vi "SubPanel_PowerConfiguration_Rev11_v4.vi"(8 "error in":errorcluster, 10 "VISAPowerInfoInputArray":T2(array[cluster]), 11 "DCPowerInformationClusterArray_Input":T1(array[cluster])) -> (0 "error out":errorcluster, 2 "VISAPowerInfoOutputArray":T2(array[cluster]), 3 "DCPowerInformationClusterArray_Output":T1(array[cluster]))   [LabVIEW 2019]
uses:
  Controls/PlotColorArray.ctl
panel:
  out "Current Numeric (A)":dbl[][](array[numeric])
  out "Voltage Numeric (V)":dbl[][](array[numeric])
  out "Voltage Waveform Array":waveform(dbl)[](graph)
  out "Current Waveform Array":waveform(dbl)[](graph)
  out "Supplies Updated?":bool
  out "DCPowerInformationClusterArray":T1(array[cluster])
  in  "Update Changes (MUST HAVE ACTIVE CHANNEL SELECTED FOR CHANGES TO BE APPLIED)":bool
  out "VISAPowerInformationClusterArray":T2(array[cluster])
  out "VISAPowerInformationClusterOutput":T3(array[cluster])
  in  "VISAPowerInformationClusterInput":T3(array[cluster])
  in  "Exit SubVI":bool
  in  "Instrument Cards (Must Reconfigure if you add new cards or change the names in NI Max)":T4(tab)
  in  "VISA resource name":refnum<visa-resource-name>
  in  "Apply Power Settings":bool
  out "POWER STATUS":bool
  in  "POWER ON":bool
  in  "Voltage Channel 1":dbl
  in  "Voltage Channel 2":dbl
  in  "Voltage Channel 3":dbl
  in  "Current Limit Channel 1":dbl
  in  "Current Limit Channel 2":dbl
  in  "Current Limit Channel 3":dbl
  out "Parameter Configuration Echo":string[][](array[string])
  out "Configuration Echo":string
  in  "Which Channels to Parallelize":u16(ring) items=["I1+I2", "ALL", "I2+I3"]
  in  "Combination Scheme":u16(ring) items=["OFF", "SERIES", "PARALLEL"]
  in  "voltage level channel 0":dbl format="%.6p"
  in  "voltage level channel 1":dbl format="%.6p"
  in  "voltage level channel 2":dbl format="%.6p"
  in  "voltage level channel 3":dbl format="%.6p"
  in  "voltage level channel 4":dbl format="%.6p"
  in  "voltage level channel 5":dbl format="%.6p"
  in  "voltage level channel 6":dbl format="%.6p"
  in  "voltage level channel 7":dbl format="%.6p"
  in  "voltage level channel 8":dbl format="%.6p"
  in  "voltage level channel 9":dbl format="%.6p"
  in  "voltage level channel 10":dbl format="%.6p"
  in  "voltage level channel 11":dbl format="%.6p"
  in  "voltage level channel 12":dbl format="%.6p"
  in  "voltage level channel 13":dbl format="%.6p"
  in  "voltage level channel 14":dbl format="%.6p"
  in  "voltage level channel 15":dbl format="%.6p"
  in  "voltage level channel 16":dbl format="%.6p"
  in  "voltage level channel 17":dbl format="%.6p"
  in  "voltage level channel 18":dbl format="%.6p"
  in  "voltage level channel 19":dbl format="%.6p"
  in  "voltage level channel 20":dbl format="%.6p"
  in  "voltage level channel 21":dbl format="%.6p"
  in  "voltage level channel 22":dbl format="%.6p"
  in  "voltage level channel 23":dbl format="%.6p"
  in  "Active Channel 0":bool
  in  "Active Channel 1":bool
  in  "Active Channel 2":bool
  in  "Active Channel 3":bool
  in  "Active Channel 4":bool
  in  "Active Channel 5":bool
  in  "Active Channel 6":bool
  in  "Active Channel 7":bool
  in  "Active Channel 8":bool
  in  "Active Channel 9":bool
  in  "Active Channel 10":bool
  in  "Active Channel 11":bool
  in  "Active Channel 12":bool
  in  "Active Channel 13":bool
  in  "Active Channel 14":bool
  in  "Active Channel 15":bool
  in  "Active Channel 16":bool
  in  "Active Channel 17":bool
  in  "Active Channel 18":bool
  in  "Active Channel 19":bool
  in  "Active Channel 20":bool
  in  "Active Channel 21":bool
  in  "Active Channel 22":bool
  in  "Active Channel 23":bool
  in  "Channel Name 0":string="NULL0"
  in  "Channel Name 1":string="NULL1"
  in  "Channel Name 2":string="NULL2"
  in  "Channel Name 3":string="NULL3"
  in  "Channel Name 4":string="NULL4"
  in  "Channel Name 5":string="NULL5"
  in  "Channel Name 6":string="NULL6"
  in  "Channel Name 7":string="NULL7"
  in  "Channel Name 8":string="NULL8"
  in  "Channel Name 9":string="NULL9"
  in  "Channel Name 10":string="NULL10"
  in  "Channel Name 11":string="NULL11"
  in  "Channel Name 12":string="NULL12"
  in  "Channel Name 13":string="NULL13"
  in  "Channel Name 14":string="NULL14"
  in  "Channel Name 15":string="NULL15"
  in  "Channel Name 16":string="NULL16"
  in  "Channel Name 17":string="NULL17"
  in  "Channel Name 18":string="NULL18"
  in  "Channel Name 19":string="NULL19"
  in  "Channel Name 20":string="NULL20"
  in  "Channel Name 21":string="NULL21"
  in  "Channel Name 22":string="NULL22"
  in  "Channel Name 23":string="NULL23"
  in  "Apply Power Settings":bool
  in  "Aperture Time (s)":dbl=0.0001
  in  "Measure Record Length":i32=1000000
  in  "current limit (A)":dbl=0.05
  out "All Channel Numbers Array":string[](array[string])=["0", "1", "2", "3", "4", "5", "6", "7", "8", "9", "10", "11", "12", "13", "14", "15", "16", "17", "18", "19", "20", "21", "22", "23"]
  out "Active Channels Indicator":bool[](array[boolean])
  out "Voltage Array":dbl[](array[numeric])
  out "Active Channel Numbers Array":string[](array[string])
  out "Active Channel Voltage Array":dbl[](array[numeric])
  out "Active Channel Names Array":string[](array[string])
  in  "voltage level channel 0":dbl=1.0 format="%.6p"
  in  "Active Channel 0":bool
  in  "Apply Power Settings":bool
  in  "Channel Name 0":string="NULL_0_slot16"
  out "Active Channel Voltage Array":dbl[](array[numeric])
  out "Active Channels Indicator":bool[](array[boolean])
  out "Voltage Array":dbl[](array[numeric])=[1.0]
  out "Active Channel Names Array":string[](array[string])
  out "Active Channel Numbers Array":string[](array[string])
  out "All Channel Numbers Array":string[](array[string])=["0"]
  in  "current limit (A)":dbl=3.0
  in  "Measure Record Length":i32=1000000
  in  "Aperture Time (s)":dbl=0.001
  in  "Apply Power Settings":bool
  in  "Aperture Time (s)":dbl=0.001
  in  "Measure Record Length":i32=1000000
  in  "current limit (A)":dbl=3.0
  in  "Active Channel 0":bool
  in  "voltage level channel 24":dbl=2.0 caption="voltage level channel 0" format="%.6p"
  in  "Channel Name 0":string="NULL_0_slot_16"
  out "Active Channel Names Array":string[](array[string])
  out "Active Channel Voltage Array":dbl[](array[numeric])
  out "Active Channel Numbers Array":string[](array[string])
  out "Voltage Array":dbl[](array[numeric])=[2.0]
  out "Active Channels Indicator":bool[](array[boolean])
  out "All Channel Numbers Array":string[](array[string])=["0"]
  out "Active Channel Names Array":string[](array[string])
  out "Active Channel Voltage Array":dbl[](array[numeric])
  out "Active Channel Numbers Array":string[](array[string])
  out "Voltage Array":dbl[](array[numeric])=[3.0]
  out "All Channel Numbers Array":string[](array[string])=["0"]
  out "Active Channels Indicator":bool[](array[boolean])
  in  "voltage level channel 25":dbl=3.0 caption="voltage level channel 0" format="%.6p"
  in  "Active Channel 0":bool
  in  "Channel Name 0":string="NULL_0_slot16"
  in  "Apply Power Settings":bool
  in  "Aperture Time (s)":dbl=0.001
  in  "Measure Record Length":i32=1000000
  in  "current limit (A)":dbl=3.0
  out "DCPowerInformationClusterOutput":T5(array[cluster])
  in  "DCPowerInformationClusterInput":T5(array[cluster])
  in  "ColorPalette":T6=[16711686, 65351, 8978420, 14474240, 16139007, 16752640, 8958719, 16758973, 16777215, 46792, 11992992, 12961221, 16763690, 12600063, 16711835, 2953983, 40796, 13111296, 13352613, 9221011, 12964076, 12819897, 65442, 16776704, 14540253, 16740729, 10658047, 10813344, 16753521, 13413843, 8691115, 10339240, 14401205, 16746704, 7467519, 16775978, 13872558, 11387603, 13354405, 10420227, 13107364, 4060, 35208, 11817216, 7566080, 40796, 7539456, 2837073, 6372186, 7499083, 10648702, 16757152]
  # "Background Information (Important)\nThis subvi has tabs that allow you to configure different power instruments. There are two options: VISA instruments or DC Power instruments. DC Power instruments are inside of the tester, visa instruments are external. If DCPower instruments are switched out, they will need to be reconfigured within the backend of this code (instructions pending). You are able to identify which channels you want to active, their individual voltage levels and the desired \"name\" of the channel (i.e. if you want channel 0 to be known at the \"ADMV1013_3p3V\" or \"GoodEnough\", you write it here). For the entire instrument, you can determine its capture rate (aperture time) or the current limit. I advise you do NOT alter the \"Measure Record Length\" as this is only if there are issues with the program. Shouldn't ever exceed this value. You apply the settings and they will be echoed back in each tab along with the array above. Multiple instruments can be configured and will show up as separate array elements\n\n\nInstructions (More Important):\n\nSelect instrument of interest (VISA KEITHLEY 2230G-30-6, PXIe-4163, and PXIe-4139 are the ones currently available). \n\n\nFOR DCPOWER INSTRUMENTS (PXI or PXIe)\n\nPress \"Active Channel #\" to select which channels you want to have power applied \n\nType in voltage level in \"Voltage level channel #\"\n\nType in desired channel name in \"Channel Name #\"\n\nType the measurement speed (suggest .0001) in aperture time\n\nType the current limit in \"current limit\"\n\nPress \"Apply Power Settings\" and review the echoed outputs within the tab and in the instrument array above the tabs.\n\nRepeat this process for other instruments\n\n\n\nFOR VISA INSTRUMENTS (NOT PXI or PXIe), note that it is case by case for instruments\n\nSelect resource name (you must know which one it is)\n\nPower on device if using it\n\nApply voltage settings \n\nApply current limits for each channel\n\nSelect which channels you will parallelize if at all\n\nSelect which combination scheme you will apply: OFF (individual channels), SERIES (Channel 1 and 2 in series), PARALLEL (I1 + I2, ALL, I2 + I3)\n\nFOR COMBINATIONS: for a combination scheme you choose, you only apply changes to the first channel of each. example: if you make the system series configuration, you only type you voltage information (i.e. 60V) into channel 1 and the current limit information into channel 1 but channel 3 is still independent of these\n\n\nPress \"Apply Powe Settings\" when complete\n\nReview the echoed values along with the instrument array above"
  # "All Voltage Level Channels are in Volts"
  # "Don't press enter when typing in strings. Just click out of it"
  # "Don't press enter when typing in strings. Just click out of it"
  # "Don't press enter when typing in strings. Just click out of it"
  # "Don't press enter when typing in strings. Just click out of it"
  # "Don't press enter when typing in strings. Just click out of it"
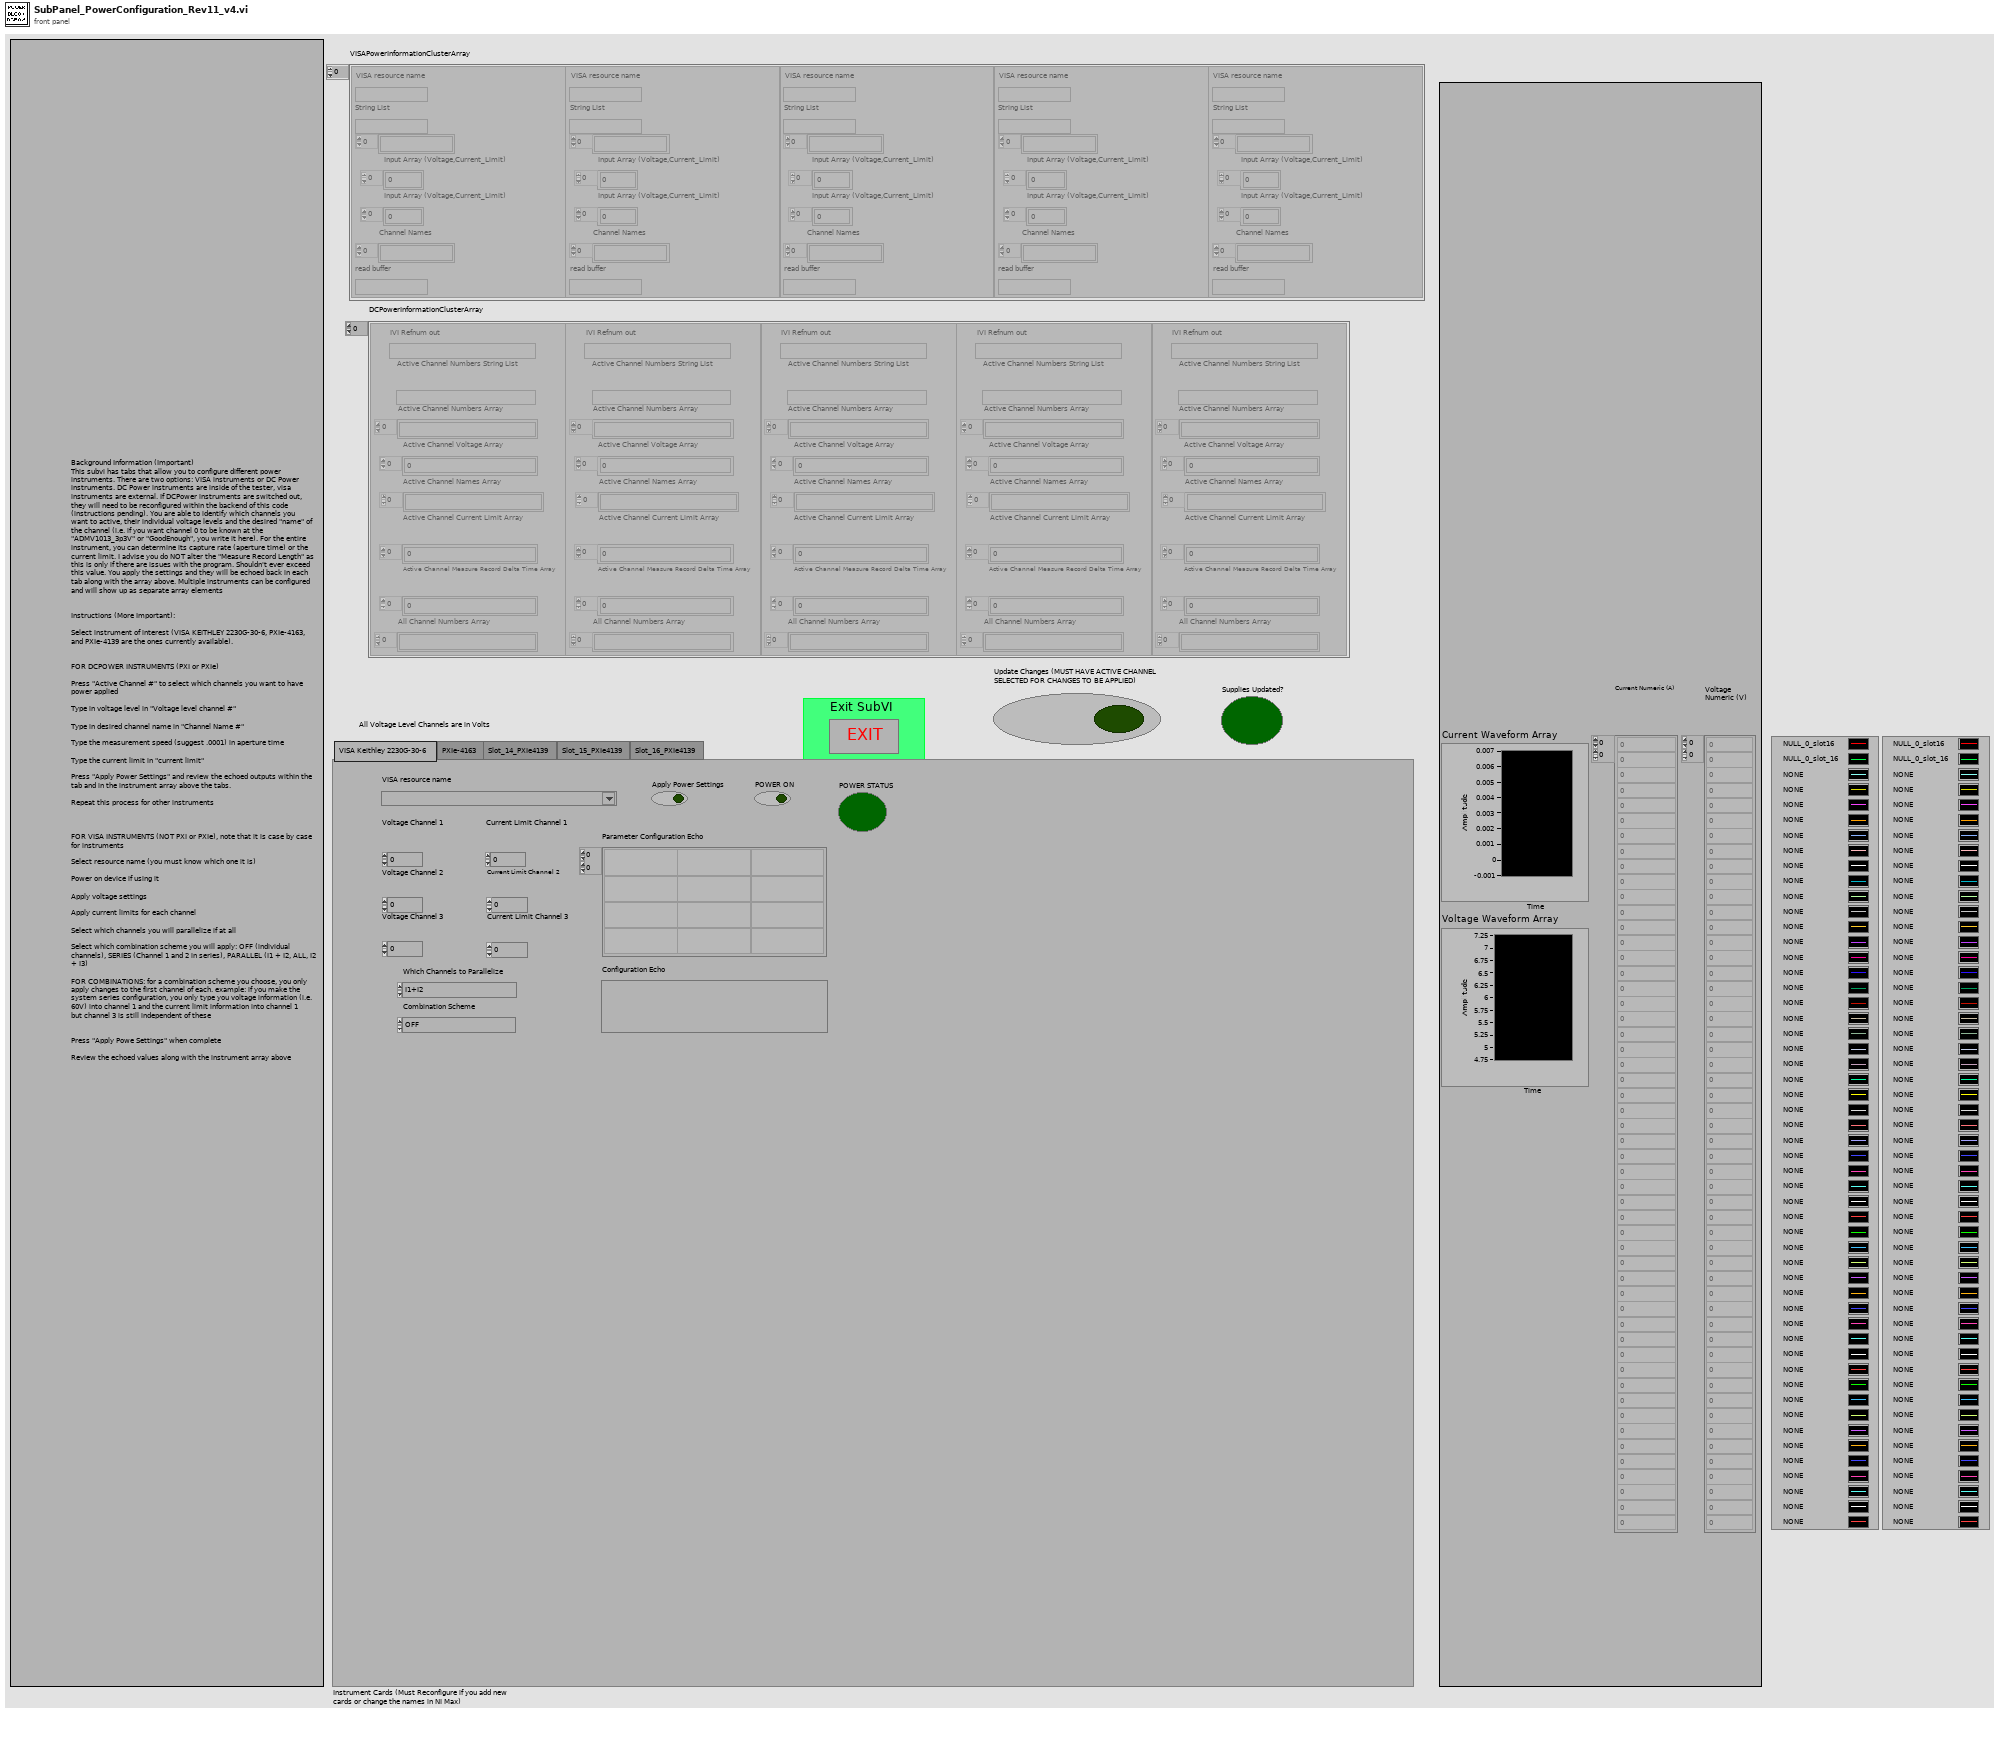
[diagram p1: front panel]
types:
  T1 = cluster{"IVI Refnum out":refnum<k15>, "Active Channel Numbers String List":string, "Active Channel Numbers Array":string[], "Active Channel Voltage Array":dbl[], "Active Channel Names Array":string[], "Active Channel Current Limit Array":dbl[], "Active Channel Measure Record Delta Time Array":dbl[], "All Channel Numbers Array":string[]}[]
  T2 = cluster{"VISA resource name":refnum<visa-resource-name>, "String List":string, string[], "Input Array (Voltage,Current_Limit)":dbl[], "Input Array (Voltage,Current_Limit)":dbl[], "Channel Names":string[], "read buffer":string}[]
  T3 = cluster{"VISA resource name":refnum<visa-resource-name>, "String List":string, string[], "Input Array (Voltage,Current_Limit)":dbl[], "Input Array (Voltage,Current_Limit)":dbl[], "Channel Names":string[]}[]
  T4 = enum32{"VISA Keithley 2230G-30-6", "PXIe-4163", "Slot_14_PXIe4139", "Slot_15_PXIe4139", "Slot_16_PXIe4139"}
  T5 = cluster{"instrument handle out":refnum<k15>, string, string[], dbl[], string[]}[]
  T6 = typedef "PlotColorArray.ctl" = u32[]
  T7 = cluster{"instrument handle out":refnum<k15>, string, string[], dbl[], string[], "Current Limit Output Array":dbl[], dbl[]}[]
  T8 = cluster{"IVI Refnum out":refnum<k15>, "Active Channel Numbers String List":string, "Active Channel Numbers Array":string[], "Active Channel Voltage Array":dbl[], "Active Channel Names Array":string[], "Active Channel Current Limit Array":dbl[], "Active Channel Measure Record Delta Time Array":dbl[], "All Channel Numbers Array":string[]}
  T9 = cluster{"IVI Refnum out":refnum<k15>, string, "voltage level channel 23":dbl, "Channel Name 23":string, "Current Limit":dbl, "Measure Record dt":dbl, string}[]
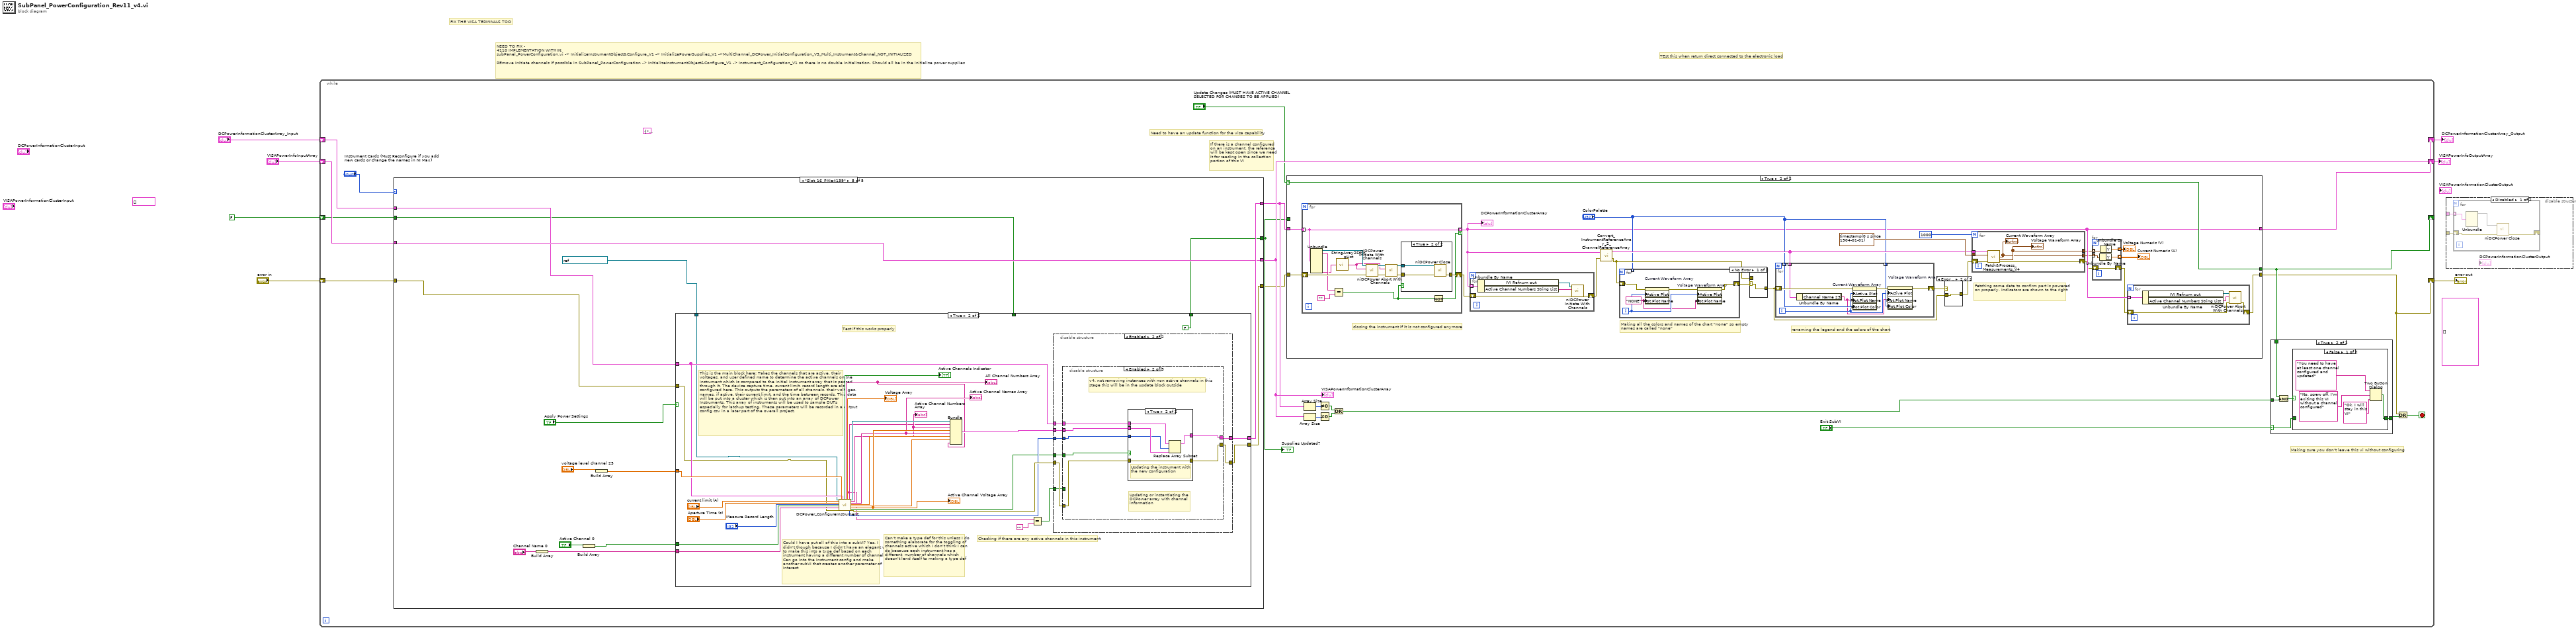
[diagram p0: block diagram]
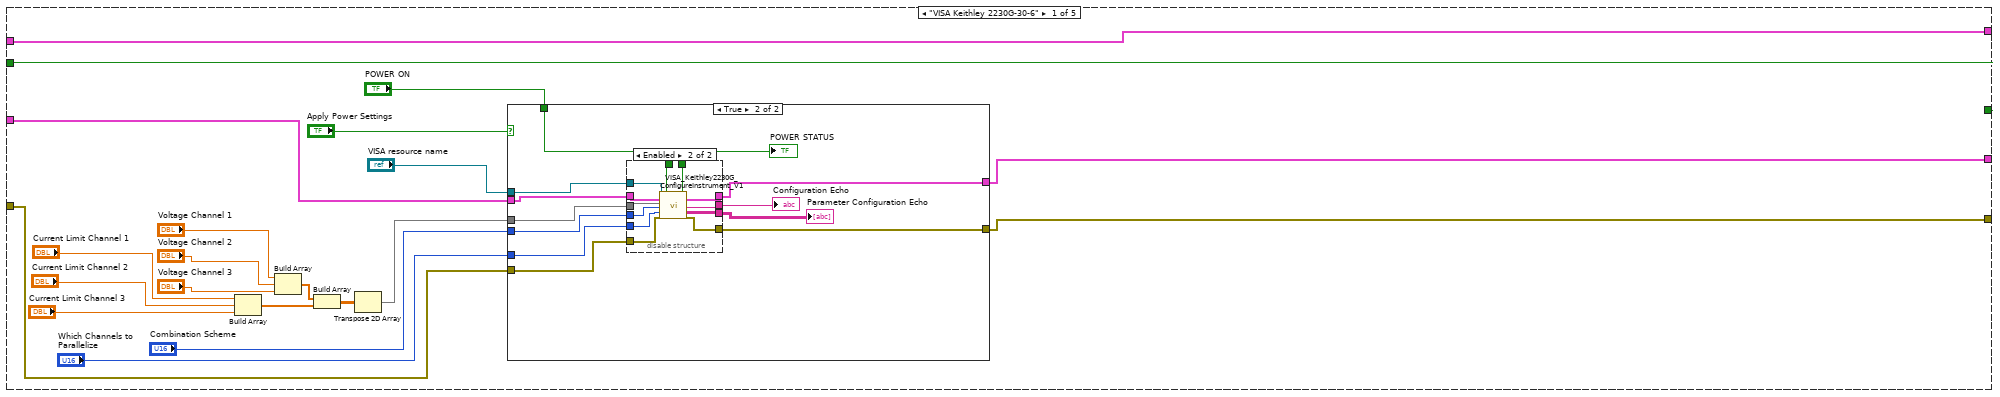
[diagram p9: hidden frame]
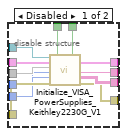
[diagram p11: hidden frame]
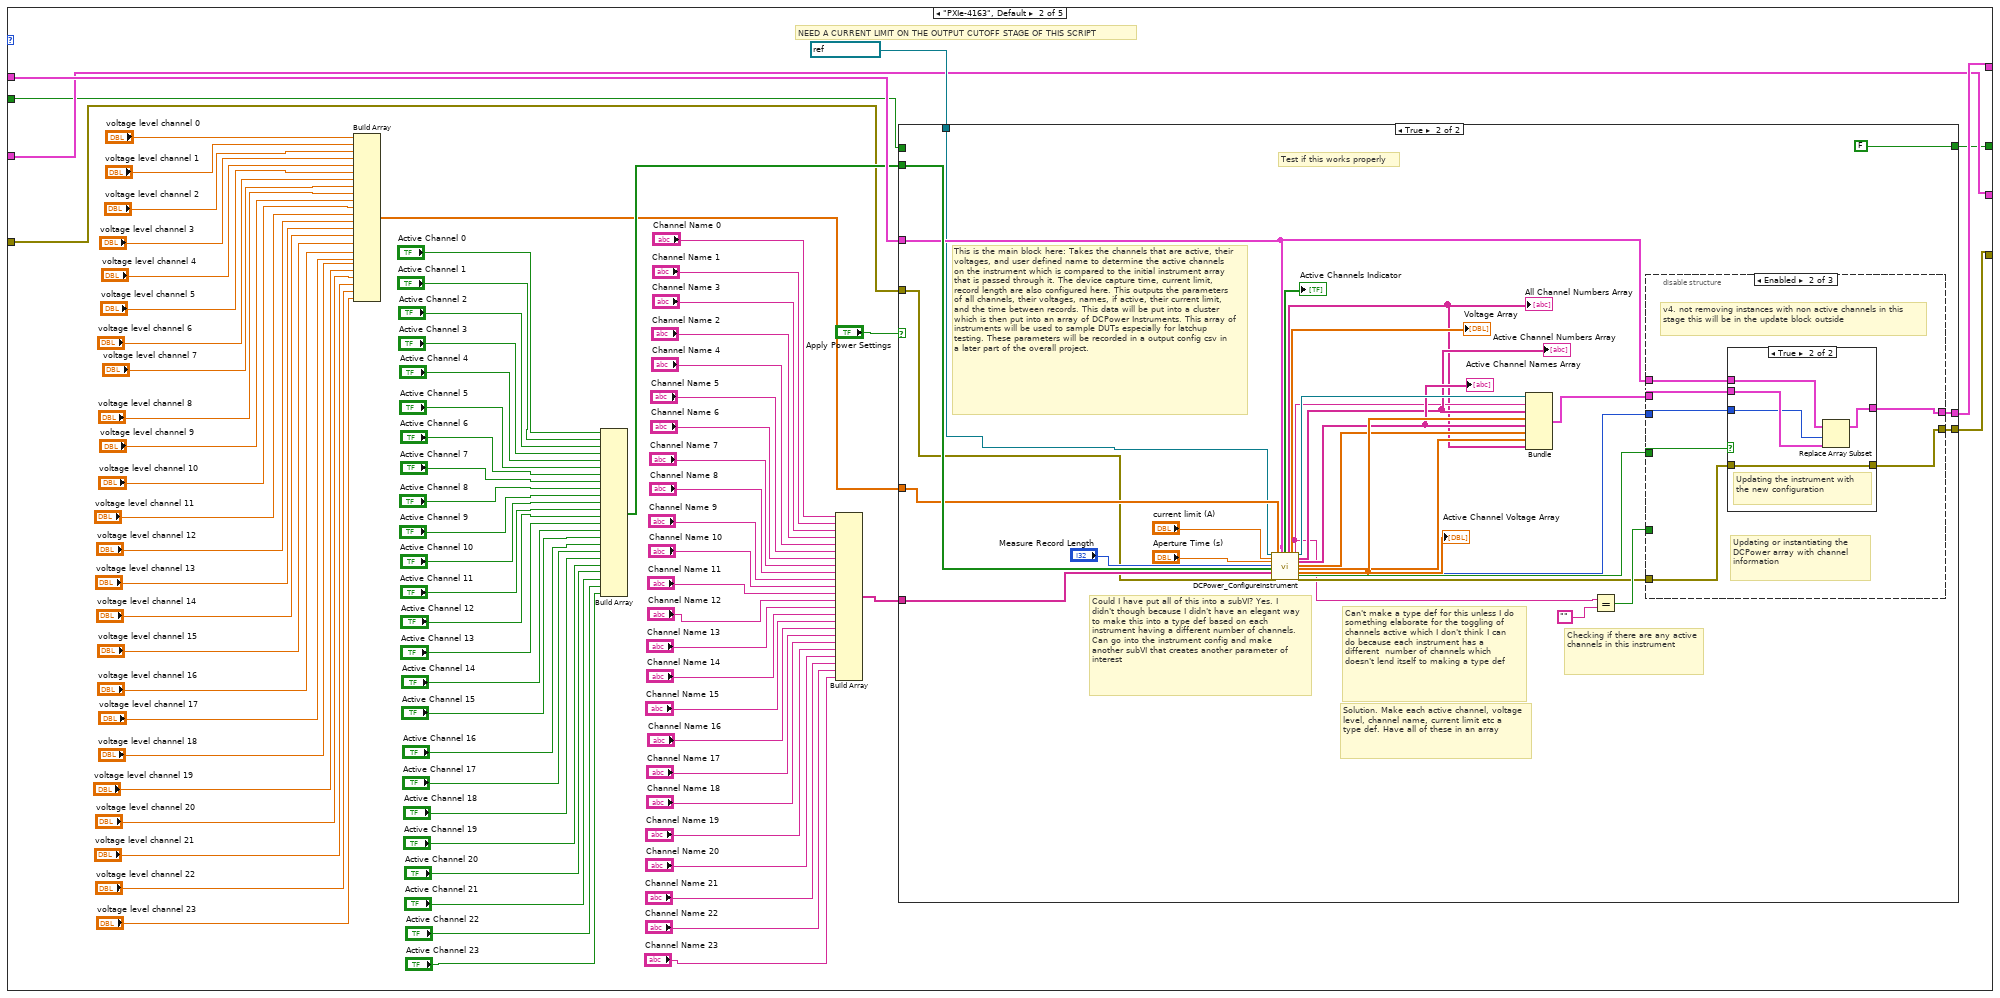
[diagram p12: hidden frame]
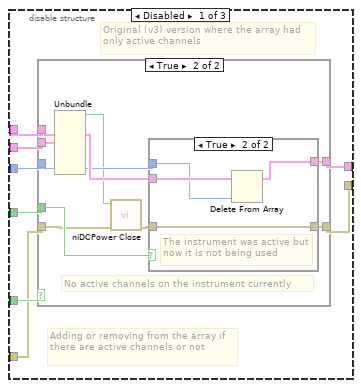
[diagram p14: hidden frame]
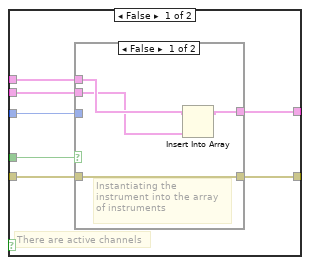
[diagram p15: hidden frame]
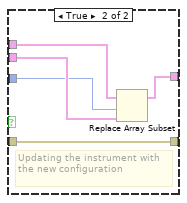
[diagram p16: hidden frame]
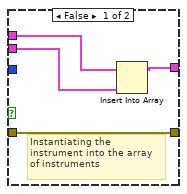
[diagram p18: hidden frame]
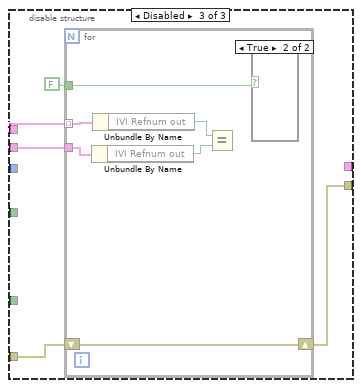
[diagram p19: hidden frame]
diagram:
  (unwired) T1 []
  (unwired) T7 [] ("DCPowerInformationClusterArray_Input")
  # "TEst this when return direct connected to the electronic load"
  # "FIX THE VISA TERMINALS TOO"
  # "NEED TO FIX - \n4110 IMPLEMENTATION WITHIN:\nsubPanel_PowerConfiguration.vi -> InitializeInstrumentObject&Configure_V1 -> InitializePowerSupplies_V1 ->MultiChannel_DCPower_InitialConfiguration_V3_Multi_Instrument&Channel_NOT_INITIALIZED\n\nREmove Initiate channels if possible in SubPanel_PowerConfiguration -> InitializeInstrumentObject&Configure_V1 -> Instrument_Configuration_V1 so there is no double initialization. Should all be in the initialize power supplies"
  n1 = while {
    shift-right: [w9] -> w3
    shift-left: "DCPowerInformationClusterArray_Input" -> [w11]
    shift-right: [w8] -> w6
    shift-left: "error in" -> [w10]
    shift-right: [w26] -> w4
    shift-left: "VISAPowerInfoInputArray" -> [w27]
    shift-right: [w12] -> _
    shift-left: FALSE -> [w13]
    stop <- w18 stop-if-true
    (unwired) T8 {"IVI Refnum out"="", "Active Channel Numbers String List"="", "Active Channel Numbers Array"=[], "Active Channel Voltage Array"=[], "Active Channel Names Array"=[], "Active Channel Current Limit Array"=[], "Active Channel Measure Record Delta Time Array"=[], "All Channel Numbers Array"=[]} ("output cluster")
    # "Making sure you don't leave this vi without configuring"
    # "Need to have an update function for the visa capability"
    # "If there is a channel configured on an instrument, the reference will be kept open since we need it for reading in the collection portion of this VI"
    n2 = case shown="\"Slot_16_PXIe4139\"" "Instrument Cards (Must Reconfigure if you add new cards or change the names in NI Max)" {
      tunnel: w11 -> [w138 w190 w363 w522 w681]
      tunnel: w10 -> [w126 w186 w371 w530 w689]
      tunnel: [w123 w185 w365 w524 w683] -> w15
      tunnel: [w138 w184 w366 w525 w684] -> w17
      tunnel: w27 -> [w139 w183 w364 w523 w682]
      tunnel: [w122 w183 w364 w523 w682] -> w26
      tunnel: [w121 w181 w362 w520 w680] -> w14
      tunnel: w13 -> [w121 w180 w361 w521 w679]
      frame "VISA Keithley 2230G-30-6" {
        n3 = Build Array("Current Limit Channel 1", "Current Limit Channel 2", "Current Limit Channel 3") -> (w136:dbl[])
        n4 = Build Array("Voltage Channel 1", "Voltage Channel 2", "Voltage Channel 3") -> (w135:dbl[])
        n5 = Build Array(w135, w136) -> (w137:dbl[][])
        n6 = Transpose 2D Array(2D array=w137) -> (transposed array=w127:dbl[][])
        n7 = case shown="True" "Apply Power Settings" {
          tunnel: "VISA resource name" -> [_ w155]
          tunnel: w139 -> [w142 w154]
          tunnel: "POWER ON" -> [_ w153]
          tunnel: w127 -> [_ w152]
          tunnel: w126 -> [w143 w151]
          tunnel: "Which Channels to Parallelize" -> [_ w150]
          tunnel: "Combination Scheme" -> [_ w149]
          tunnel: [w142 w145] -> w122
          tunnel: [w143 w144] -> w123
          frame False {
          }
          frame True {
            n8 = disable-structure shown="Enabled" {
              disable-tunnel: w155 -> [w167 w177]
              disable-tunnel: w154 -> [w166 w176]
              disable-tunnel: w153 -> [w165 w178]
              disable-tunnel: w152 -> [w164 w175]
              disable-tunnel: w151 -> [w163 w172]
              disable-tunnel: w150 -> [w162 w173]
              disable-tunnel: w149 -> [w161 w174]
              disable-tunnel: [w160 w179] -> w148
              disable-tunnel: [w159 w170] -> w147
              disable-tunnel: [w158 w169] -> w146
              disable-tunnel: [w157 w171] -> w145
              disable-tunnel: [w156 w168] -> w144
              frame Disabled {
                n9 = call "Initialize_VISA_PowerSupplies_Keithley2230G_V1.vi"("VISA resource name"=w167, "VISAPowerInfoInputArray"=w166, "Input Array (Voltage,Current_Limit)"=w164, "Combination Scheme"=w161, "Which Channels to Parallelize"=w162, "error in"=w163, "POWER STATUS IN"=w165) -> ("POWER STATUS OUT"=w160:bool, "VISAPowerInfoOutputArray"=w157:T2, "Configuration Echo"=w159:string, "Parameter Configuration Echo"=w158:string[][], "error out"=w156:errorcluster)  [unwired: 8 in]
              }
              frame Enabled {
                n10 = call "VISA_Keithley2230G_ConfigureInstrument_V1.vi"("VISA resource name"=w177, "VISAPowerInfoInputArray"=w176, "Input Array (Voltage,Current_Limit)"=w175, "Combination Scheme"=w174, "Which Channels to Parallelize"=w173, "error in"=w172, "POWER STATUS IN"=w178) -> ("POWER STATUS OUT"=w179:bool, "VISAPowerInfoOutputArray"=w171:T2, "Configuration Echo"=w170:string, "Parameter Configuration Echo"=w169:string[][], "error out"=w168:errorcluster)  [unwired: 8 in]
              }
            }
            "POWER STATUS" <- w148
            "Configuration Echo" <- w147
            "Parameter Configuration Echo" <- w146
          }
        }
      }
      frame "PXIe-4163", Default {
        # "NEED A CURRENT LIMIT ON THE OUTPUT CUTOFF STAGE OF THIS SCRIPT"
        n11 = Build Array("voltage level channel 0", "voltage level channel 1", "voltage level channel 2", "voltage level channel 3", "voltage level channel 4", "voltage level channel 5", "voltage level channel 6", "voltage level channel 7", "voltage level channel 8", "voltage level channel 9", "voltage level channel 10", "voltage level channel 11", "voltage level channel 12", "voltage level channel 13", "voltage level channel 14", "voltage level channel 15", "voltage level channel 16", "voltage level channel 17", "voltage level channel 18", "voltage level channel 19", "voltage level channel 20", "voltage level channel 21", "voltage level channel 22", "voltage level channel 23") -> (w182:dbl[])
        n12 = Build Array("Active Channel 0", "Active Channel 1", "Active Channel 2", "Active Channel 3", "Active Channel 4", "Active Channel 5", "Active Channel 6", "Active Channel 7", "Active Channel 8", "Active Channel 9", "Active Channel 10", "Active Channel 11", "Active Channel 12", "Active Channel 13", "Active Channel 14", "Active Channel 15", "Active Channel 16", "Active Channel 17", "Active Channel 18", "Active Channel 19", "Active Channel 20", "Active Channel 21", "Active Channel 22", "Active Channel 23") -> (w188:bool[])
        n13 = Build Array("Channel Name 0", "Channel Name 1", "Channel Name 3", "Channel Name 2", "Channel Name 4", "Channel Name 5", "Channel Name 6", "Channel Name 7", "Channel Name 8", "Channel Name 9", "Channel Name 10", "Channel Name 11", "Channel Name 12", "Channel Name 13", "Channel Name 14", "Channel Name 15", "Channel Name 16", "Channel Name 17", "Channel Name 18", "Channel Name 19", "Channel Name 20", "Channel Name 21", "Channel Name 22", "Channel Name 23") -> (w187:string[])
        n14 = case shown="True" "Apply Power Settings" {
          tunnel: w190 -> [w266 w279]
          tunnel: refnum<k15> "PXIe-4163" ("resource name") -> [_ w267]
          tunnel: w188 -> [_ w294]
          tunnel: w187 -> [_ w292]
          tunnel: w186 -> [w265 w268]
          tunnel: [w265 w277] -> w185
          tunnel: [w266 w276] -> w184
          tunnel: w182 -> [_ w293]
          tunnel: [w264 FALSE] -> w181
          tunnel: w180 -> [w264 _]
          frame False {
          }
          frame True {
            # "Solution. Make each active channel, voltage level, channel name, current limit etc a type def. Have all of these in an array"
            # "This is the main block here: Takes the channels that are active, their voltages, and user defined name to determine the active channels on the instrument which is compared to the initial instrument array that is passed through it. The device capture time, current limit, record length are also configured here. This outputs the parameters of all channels, their voltages, names, if active, their current limit, and the time between records. This data will be put into a cluster which is then put into an array of DCPower Instruments. This array of instruments will be used to sample DUTs especially for latchup testing. These parameters will be recorded in a output config csv in a later part of the overall project."
            # "Checking if there are any active channels in this instrument"
            # "Could I have put all of this into a subVI? Yes. I didn't though because I didn't have an elegant way to make this into a type def based on each instrument having a different number of channels. Can go into the instrument config and make another subVI that creates another parameter of interest"
            # "Can't make a type def for this unless I do something elaborate for the toggling of channels active which I don't think I can do because each instrument has a different  number of channels which doesn't lend itself to making a type def"
            # "Test if this works properly"
            n15 = call "DCPower_ConfigureInstrument.vi"("IVI Refnum in"=w267, "current limit"="current limit (A)", "Aperture Time"="Aperture Time (s)", "Measure Record Length"="Measure Record Length", "Active Channels Input"=w294, "Channel Name Array"=w292, "error in (no error)"=w268, "Voltage Array Input"=w293, "DCPowerInformationClusterArray_Input"=w279) -> ("Active Channels Indicator"=→"Active Channels Indicator":bool[], "All Channel Numbers Array"=w270:string[], "Total Voltage Indicator Array"=→"Voltage Array":dbl[], "Active Channel Numbers String List"=w271:string, "IVI Ref index"=w275:i32, "IVI Refnum out"=w287:refnum<k15>, "Active Channel Numbers Array"=w273:string[], "Active Channel Names Array"=w285:string[], "Active Channel Current Limit Array"=w284:dbl[], "Active Channel Measure Record Delta Time Array"=w283:dbl[], "Active Channel Voltage Array"=w286:dbl[], "IVI Ref Present?"=w274:bool, "error out"=w278:errorcluster)  [unwired: 5 in, 1 out]
            "All Channel Numbers Array" <- w270
            "Active Channel Numbers Array" <- w273
            "Active Channel Names Array" <- w285
            "Active Channel Voltage Array" <- w286
            n16 = Bundle("IVI Refnum out"=w287, "Active Channel Numbers String List"=w271, "Active Channel Numbers Array"=w273, "Active Channel Voltage Array"=w286, "Active Channel Names Array"=w285, "Active Channel Current Limit Array"=w284, "Active Channel Measure Record Delta Time Array"=w283, "All Channel Numbers Array"=w270) -> (w280:T8)  [unwired: 1 in]
            n17 = Equal?(x=w271, y="") -> (x = y?=w281:bool)
            n18 = disable-structure shown="Enabled" {
              disable-tunnel: w281 -> [w302 _ _]
              disable-tunnel: w280 -> [w301 w340 w351]
              disable-tunnel: w279 -> [w300 w339 w354]
              disable-tunnel: w278 -> [w299 w338 w352]
              disable-tunnel: [w298 w337 w353] -> w277
              disable-tunnel: [w297 w336 _] -> w276
              disable-tunnel: w275 -> [w296 w335 _]
              disable-tunnel: w274 -> [w295 w334 _]
              frame Disabled {
                # "Original (v3) version where the array had only active channels"
                # "Adding or removing from the array if there are active channels or not"
                n19 = case shown="True" w302 {
                  tunnel: w295 -> [w309 w326]
                  tunnel: [w308 w323] -> w297
                  tunnel: [w307 w324] -> w298
                  tunnel: w299 -> [w306 w321]
                  tunnel: w296 -> [w305 w325]
                  tunnel: w301 -> [w304 w319]
                  tunnel: w300 -> [w303 w327]
                  frame False {
                    # "There are active channels"
                    n20 = case shown="False" w309 {
                      tunnel: w303 -> [w312 w318]
                      tunnel: w304 -> [w311 w317]
                      tunnel: w305 -> [_ w316]
                      tunnel: w306 -> [w313 w315]
                      tunnel: [w313 w315] -> w307
                      tunnel: [w310 w314] -> w308
                      frame False {
                        # "Instantiating the instrument into the array of instruments"
                        n21 = Insert Into Array(array=w312, new element=w311) -> (w310:T1)  [unwired: 1 in]
                      }
                      frame True {
                        # "Updating the instrument with the new configuration"
                        n22 = Replace Array Subset(array=w318, new element=w317, index=w316) -> (w314:T1)
                      }
                    }
                  }
                  frame True {
                    # "No active channels on the instrument currently"
                    n23 = Unbundle(w319) -> ("IVI Refnum out"=w322:refnum<k15>)  [unwired: 7 out]
                    n24 = call <instrlib>:"niDCPower Close.vi"("error in (no error)"=w321, "instrument handle"=w322) -> ("error out"=w320:errorcluster)  [unwired: 9 in]
                    n25 = case shown="True" w326 {
                      tunnel: w327 -> [w329 w333]
                      tunnel: w325 -> [_ w332]
                      tunnel: [w328 w331] -> w324
                      tunnel: w320 -> [w328 w331]
                      tunnel: [w329 w330] -> w323
                      frame False {
                        # "The instrument wasn't active and it is still not being used"
                      }
                      frame True {
                        # "The instrument was active but now it is not being used"
                        n26 = Delete From Array(array=w333, index=w332) -> (array with subset deleted=w330:T1)  [unwired: 1 in, 1 out]
                      }
                    }
                  }
                }
              }
              frame Enabled {
                # "v4. not removing instances with non active channels in this stage this will be in the update block outside"
                # "Updating or instantiating the DCPower array with channel information"
                n27 = case shown="True" w334 {
                  tunnel: w339 -> [w343 w349]
                  tunnel: w340 -> [w342 w348]
                  tunnel: w335 -> [_ w347]
                  tunnel: w338 -> [w344 w346]
                  tunnel: [w344 w346] -> w337
                  tunnel: [w341 w345] -> w336
                  frame False {
                    # "Instantiating the instrument into the array of instruments"
                    n28 = Insert Into Array(array=w343, new element=w342) -> (w341:T1)  [unwired: 1 in]
                  }
                  frame True {
                    # "Updating the instrument with the new configuration"
                    n29 = Replace Array Subset(array=w349, new element=w348, index=w347) -> (w345:T1)
                  }
                }
              }
              frame Disabled {
                n30 = for {
                  tunnel: w354 -> [w360] mode=indexing
                  shift-right: [w359] -> w353
                  shift-left: w352 -> [w359]
                  tunnel: w351 -> [w357]
                  tunnel: FALSE -> [w355]
                  n31 = Unbundle By Name(w357) -> ("IVI Refnum out"=w356:refnum<k15>)
                  n32 = Unbundle By Name(w360) -> ("IVI Refnum out"=w358:refnum<k15>)
                  n33 = Equal?(x=w358, y=w356) -> ()  [unwired: 1 out]
                  n34 = case shown="True" w355 {
                    frame False {
                    }
                    frame True {
                    }
                  }
                }
              }
            }
          }
        }
      }
      frame "Slot_14_PXIe4139" {
        n35 = Build Array("Channel Name 0") -> (w368:string[])
        n36 = Build Array("Active Channel 0") -> (w369:bool[])
        n37 = Build Array("voltage level channel 0") -> (w370:dbl[])
        n38 = case shown="True" "Apply Power Settings" {
          tunnel: w363 -> [w378 w391]
          tunnel: refnum<k15> "Slot_14_PXIe4139" ("resource name") -> [_ w380]
          tunnel: w369 -> [_ w406]
          tunnel: w368 -> [_ w404]
          tunnel: w371 -> [w377 w379]
          tunnel: [w377 w389] -> w365
          tunnel: [w378 w388] -> w366
          tunnel: w370 -> [_ w405]
          tunnel: [w376 FALSE] -> w362
          tunnel: w361 -> [w376 _]
          frame False {
          }
          frame True {
            # "This is the main block here: Takes the channels that are active, their voltages, and user defined name to determine the active channels on the instrument which is compared to the initial instrument array that is passed through it. The device capture time, current limit, record length are also configured here. This outputs the parameters of all channels, their voltages, names, if active, their current limit, and the time between records. This data will be put into a cluster which is then put into an array of DCPower Instruments. This array of instruments will be used to sample DUTs especially for latchup testing. These parameters will be recorded in a output config csv in a later part of the overall project."
            # "Checking if there are any active channels in this instrument"
            # "Could I have put all of this into a subVI? Yes. I didn't though because I didn't have an elegant way to make this into a type def based on each instrument having a different number of channels. Can go into the instrument config and make another subVI that creates another parameter of interest"
            # "Can't make a type def for this unless I do something elaborate for the toggling of channels active which I don't think I can do because each instrument has a different  number of channels which doesn't lend itself to making a type def"
            # "Test if this works properly"
            n39 = call "DCPower_ConfigureInstrument.vi"("IVI Refnum in"=w380, "current limit"="current limit (A)", "Aperture Time"="Aperture Time (s)", "Measure Record Length"="Measure Record Length", "Active Channels Input"=w406, "Channel Name Array"=w404, "error in (no error)"=w379, "Voltage Array Input"=w405, "DCPowerInformationClusterArray_Input"=w391) -> ("Active Channels Indicator"=→"Active Channels Indicator":bool[], "All Channel Numbers Array"=w382:string[], "Total Voltage Indicator Array"=→"Voltage Array":dbl[], "Active Channel Numbers String List"=w383:string, "IVI Ref index"=w387:i32, "IVI Refnum out"=w399:refnum<k15>, "Active Channel Numbers Array"=w385:string[], "Active Channel Names Array"=w397:string[], "Active Channel Current Limit Array"=w396:dbl[], "Active Channel Measure Record Delta Time Array"=w395:dbl[], "Active Channel Voltage Array"=w398:dbl[], "IVI Ref Present?"=w386:bool, "error out"=w390:errorcluster)  [unwired: 5 in, 1 out]
            "All Channel Numbers Array" <- w382
            "Active Channel Numbers Array" <- w385
            "Active Channel Names Array" <- w397
            "Active Channel Voltage Array" <- w398
            n40 = Bundle("IVI Refnum out"=w399, "Active Channel Numbers String List"=w383, "Active Channel Numbers Array"=w385, "Active Channel Voltage Array"=w398, "Active Channel Names Array"=w397, "Active Channel Current Limit Array"=w396, "Active Channel Measure Record Delta Time Array"=w395, "All Channel Numbers Array"=w382) -> (w392:T8)  [unwired: 1 in]
            n41 = Equal?(x=w383, y="") -> (x = y?=w393:bool)
            n42 = disable-structure shown="Enabled" {
              disable-tunnel: w393 -> [w414 w449]
              disable-tunnel: w392 -> [w413 w452]
              disable-tunnel: w391 -> [w412 w453]
              disable-tunnel: w390 -> [w411 w448]
              disable-tunnel: [w410 w446] -> w389
              disable-tunnel: [w409 w447] -> w388
              disable-tunnel: w387 -> [w408 w451]
              disable-tunnel: w386 -> [w407 w450]
              frame Disabled {
                # "Adding or removing from the array if there are active channels or not"
                n43 = case shown="False" w414 {
                  tunnel: w407 -> [w421 w438]
                  tunnel: [w420 w435] -> w409
                  tunnel: [w419 w436] -> w410
                  tunnel: w411 -> [w418 w433]
                  tunnel: w408 -> [w417 w437]
                  tunnel: w413 -> [w416 w431]
                  tunnel: w412 -> [w415 w439]
                  frame False {
                    # "There are active channels"
                    n44 = case shown="True" w421 {
                      tunnel: w415 -> [w424 w430]
                      tunnel: w416 -> [w423 w429]
                      tunnel: w417 -> [_ w428]
                      tunnel: w418 -> [w425 w427]
                      tunnel: [w425 w427] -> w419
                      tunnel: [w422 w426] -> w420
                      frame False {
                        # "Instantiating the instrument into the array of instruments"
                        n45 = Insert Into Array(array=w424, new element=w423) -> (w422:T1)  [unwired: 1 in]
                      }
                      frame True {
                        # "Updating the instrument with the new configuration"
                        n46 = Replace Array Subset(array=w430, new element=w429, index=w428) -> (w426:T1)
                      }
                    }
                  }
                  frame True {
                    # "No active channels on the instrument currently"
                    n47 = Unbundle(w431) -> ("IVI Refnum out"=w434:refnum<k15>)  [unwired: 7 out]
                    n48 = call <instrlib>:"niDCPower Close.vi"("error in (no error)"=w433, "instrument handle"=w434) -> ("error out"=w432:errorcluster)  [unwired: 9 in]
                    n49 = case shown="False" w438 {
                      tunnel: w439 -> [w441 w445]
                      tunnel: w437 -> [_ w444]
                      tunnel: [w440 w443] -> w436
                      tunnel: w432 -> [w440 w443]
                      tunnel: [w441 w442] -> w435
                      frame False {
                        # "The instrument wasn't active and it is still not being used"
                      }
                      frame True {
                        # "The instrument was active but now it is not being used"
                        n50 = Delete From Array(array=w445, index=w444) -> (array with subset deleted=w442:T1)  [unwired: 1 in, 1 out]
                      }
                    }
                  }
                }
              }
              frame Enabled {
                n51 = disable-structure shown="Enabled" {
                  disable-tunnel: w449 -> [w461 _ _]
                  disable-tunnel: w452 -> [w460 w499 w510]
                  disable-tunnel: w453 -> [w459 w498 w513]
                  disable-tunnel: w448 -> [w458 w497 w511]
                  disable-tunnel: [w457 w496 w512] -> w446
                  disable-tunnel: [w456 w495 _] -> w447
                  disable-tunnel: w451 -> [w455 w494 _]
                  disable-tunnel: w450 -> [w454 w493 _]
                  frame Disabled {
                    # "Original (v3) version where the array had only active channels"
                    # "Adding or removing from the array if there are active channels or not"
                    n52 = case shown="False" w461 {
                      tunnel: w454 -> [w468 w485]
                      tunnel: [w467 w482] -> w456
                      tunnel: [w466 w483] -> w457
                      tunnel: w458 -> [w465 w480]
                      tunnel: w455 -> [w464 w484]
                      tunnel: w460 -> [w463 w478]
                      tunnel: w459 -> [w462 w486]
                      frame False {
                        # "There are active channels"
                        n53 = case shown="False" w468 {
                          tunnel: w462 -> [w471 w477]
                          tunnel: w463 -> [w470 w476]
                          tunnel: w464 -> [_ w475]
                          tunnel: w465 -> [w472 w474]
                          tunnel: [w472 w474] -> w466
                          tunnel: [w469 w473] -> w467
                          frame False {
                            # "Instantiating the instrument into the array of instruments"
                            n54 = Insert Into Array(array=w471, new element=w470) -> (w469:T1)  [unwired: 1 in]
                          }
                          frame True {
                            # "Updating the instrument with the new configuration"
                            n55 = Replace Array Subset(array=w477, new element=w476, index=w475) -> (w473:T1)
                          }
                        }
                      }
                      frame True {
                        # "No active channels on the instrument currently"
                        n56 = Unbundle(w478) -> ("IVI Refnum out"=w481:refnum<k15>)  [unwired: 7 out]
                        n57 = call <instrlib>:"niDCPower Close.vi"("error in (no error)"=w480, "instrument handle"=w481) -> ("error out"=w479:errorcluster)  [unwired: 9 in]
                        n58 = case shown="True" w485 {
                          tunnel: w486 -> [w488 w492]
                          tunnel: w484 -> [_ w491]
                          tunnel: [w487 w490] -> w483
                          tunnel: w479 -> [w487 w490]
                          tunnel: [w488 w489] -> w482
                          frame False {
                            # "The instrument wasn't active and it is still not being used"
                          }
                          frame True {
                            # "The instrument was active but now it is not being used"
                            n59 = Delete From Array(array=w492, index=w491) -> (array with subset deleted=w489:T1)  [unwired: 1 in, 1 out]
                          }
                        }
                      }
                    }
                  }
                  frame Enabled {
                    # "v4. not removing instances with non active channels in this stage this will be in the update block outside"
                    # "Updating or instantiating the DCPower array with channel information"
                    n60 = case shown="True" w493 {
                      tunnel: w498 -> [w502 w508]
                      tunnel: w499 -> [w501 w507]
                      tunnel: w494 -> [_ w506]
                      tunnel: w497 -> [w503 w505]
                      tunnel: [w503 w505] -> w496
                      tunnel: [w500 w504] -> w495
                      frame False {
                        # "Instantiating the instrument into the array of instruments"
                        n61 = Insert Into Array(array=w502, new element=w501) -> (w500:T1)  [unwired: 1 in]
                      }
                      frame True {
                        # "Updating the instrument with the new configuration"
                        n62 = Replace Array Subset(array=w508, new element=w507, index=w506) -> (w504:T1)
                      }
                    }
                  }
                  frame Disabled {
                    n63 = for {
                      tunnel: w513 -> [w519] mode=indexing
                      shift-right: [w518] -> w512
                      shift-left: w511 -> [w518]
                      tunnel: w510 -> [w516]
                      tunnel: FALSE -> [w514]
                      n64 = Unbundle By Name(w516) -> ("IVI Refnum out"=w515:refnum<k15>)
                      n65 = Unbundle By Name(w519) -> ("IVI Refnum out"=w517:refnum<k15>)
                      n66 = Equal?(x=w517, y=w515) -> ()  [unwired: 1 out]
                      n67 = case shown="True" w514 {
                        frame False {
                        }
                        frame True {
                        }
                      }
                    }
                  }
                }
              }
            }
          }
        }
      }
      frame "Slot_15_PXIe4139" {
        n68 = Build Array("Channel Name 0") -> (w527:string[])
        n69 = Build Array("Active Channel 0") -> (w528:bool[])
        n70 = Build Array("voltage level channel 24") -> (w529:dbl[])
        n71 = case shown="True" "Apply Power Settings" {
          tunnel: w522 -> [w537 w550]
          tunnel: refnum<k15> "Slot_15_PXIe4139" ("resource name") -> [_ w538]
          tunnel: w528 -> [_ w565]
          tunnel: w527 -> [_ w563]
          tunnel: w530 -> [w536 w539]
          tunnel: [w536 w548] -> w524
          tunnel: [w537 w547] -> w525
          tunnel: w529 -> [_ w564]
          tunnel: w521 -> [w535 _]
          tunnel: [w535 FALSE] -> w520
          frame False {
          }
          frame True {
            # "This is the main block here: Takes the channels that are active, their voltages, and user defined name to determine the active channels on the instrument which is compared to the initial instrument array that is passed through it. The device capture time, current limit, record length are also configured here. This outputs the parameters of all channels, their voltages, names, if active, their current limit, and the time between records. This data will be put into a cluster which is then put into an array of DCPower Instruments. This array of instruments will be used to sample DUTs especially for latchup testing. These parameters will be recorded in a output config csv in a later part of the overall project."
            # "Checking if there are any active channels in this instrument"
            # "Could I have put all of this into a subVI? Yes. I didn't though because I didn't have an elegant way to make this into a type def based on each instrument having a different number of channels. Can go into the instrument config and make another subVI that creates another parameter of interest"
            # "Can't make a type def for this unless I do something elaborate for the toggling of channels active which I don't think I can do because each instrument has a different  number of channels which doesn't lend itself to making a type def"
            # "Test if this works properly"
            n72 = call "DCPower_ConfigureInstrument.vi"("IVI Refnum in"=w538, "current limit"="current limit (A)", "Aperture Time"="Aperture Time (s)", "Measure Record Length"="Measure Record Length", "Active Channels Input"=w565, "Channel Name Array"=w563, "error in (no error)"=w539, "Voltage Array Input"=w564, "DCPowerInformationClusterArray_Input"=w550) -> ("Active Channels Indicator"=→"Active Channels Indicator":bool[], "All Channel Numbers Array"=w541:string[], "Total Voltage Indicator Array"=→"Voltage Array":dbl[], "Active Channel Numbers String List"=w542:string, "IVI Ref index"=w546:i32, "IVI Refnum out"=w558:refnum<k15>, "Active Channel Numbers Array"=w544:string[], "Active Channel Names Array"=w556:string[], "Active Channel Current Limit Array"=w555:dbl[], "Active Channel Measure Record Delta Time Array"=w554:dbl[], "Active Channel Voltage Array"=w557:dbl[], "IVI Ref Present?"=w545:bool, "error out"=w549:errorcluster)  [unwired: 5 in, 1 out]
            "All Channel Numbers Array" <- w541
            "Active Channel Numbers Array" <- w544
            "Active Channel Names Array" <- w556
            "Active Channel Voltage Array" <- w557
            n73 = Bundle("IVI Refnum out"=w558, "Active Channel Numbers String List"=w542, "Active Channel Numbers Array"=w544, "Active Channel Voltage Array"=w557, "Active Channel Names Array"=w556, "Active Channel Current Limit Array"=w555, "Active Channel Measure Record Delta Time Array"=w554, "All Channel Numbers Array"=w541) -> (w551:T8)  [unwired: 1 in]
            n74 = Equal?(x=w542, y="") -> (x = y?=w552:bool)
            n75 = disable-structure shown="Enabled" {
              disable-tunnel: w552 -> [w573 w607]
              disable-tunnel: w551 -> [w572 w611]
              disable-tunnel: w550 -> [w571 w612]
              disable-tunnel: w549 -> [w570 w608]
              disable-tunnel: [w569 w606] -> w548
              disable-tunnel: [w568 w605] -> w547
              disable-tunnel: w546 -> [w567 w610]
              disable-tunnel: w545 -> [w566 w609]
              frame Disabled {
                # "Adding or removing from the array if there are active channels or not"
                n76 = case shown="False" w573 {
                  tunnel: w566 -> [w580 w597]
                  tunnel: [w579 w594] -> w568
                  tunnel: [w578 w595] -> w569
                  tunnel: w570 -> [w577 w592]
                  tunnel: w567 -> [w576 w596]
                  tunnel: w572 -> [w575 w590]
                  tunnel: w571 -> [w574 w598]
                  frame False {
                    # "There are active channels"
                    n77 = case shown="True" w580 {
                      tunnel: w574 -> [w583 w589]
                      tunnel: w575 -> [w582 w588]
                      tunnel: w576 -> [_ w587]
                      tunnel: w577 -> [w584 w586]
                      tunnel: [w584 w586] -> w578
                      tunnel: [w581 w585] -> w579
                      frame False {
                        # "Instantiating the instrument into the array of instruments"
                        n78 = Insert Into Array(array=w583, new element=w582) -> (w581:T1)  [unwired: 1 in]
                      }
                      frame True {
                        # "Updating the instrument with the new configuration"
                        n79 = Replace Array Subset(array=w589, new element=w588, index=w587) -> (w585:T1)
                      }
                    }
                  }
                  frame True {
                    # "No active channels on the instrument currently"
                    n80 = Unbundle(w590) -> ("IVI Refnum out"=w593:refnum<k15>)  [unwired: 7 out]
                    n81 = call <instrlib>:"niDCPower Close.vi"("error in (no error)"=w592, "instrument handle"=w593) -> ("error out"=w591:errorcluster)  [unwired: 9 in]
                    n82 = case shown="False" w597 {
                      tunnel: w598 -> [w600 w604]
                      tunnel: w596 -> [_ w603]
                      tunnel: [w599 w602] -> w595
                      tunnel: w591 -> [w599 w602]
                      tunnel: [w600 w601] -> w594
                      frame False {
                        # "The instrument wasn't active and it is still not being used"
                      }
                      frame True {
                        # "The instrument was active but now it is not being used"
                        n83 = Delete From Array(array=w604, index=w603) -> (array with subset deleted=w601:T1)  [unwired: 1 in, 1 out]
                      }
                    }
                  }
                }
              }
              frame Enabled {
                n84 = disable-structure shown="Enabled" {
                  disable-tunnel: w607 -> [w620 _ _]
                  disable-tunnel: w611 -> [w619 w658 w669]
                  disable-tunnel: w612 -> [w618 w657 w672]
                  disable-tunnel: w608 -> [w617 w656 w670]
                  disable-tunnel: [w616 w655 w671] -> w606
                  disable-tunnel: [w615 w654 _] -> w605
                  disable-tunnel: w610 -> [w614 w653 _]
                  disable-tunnel: w609 -> [w613 w652 _]
                  frame Disabled {
                    # "Original (v3) version where the array had only active channels"
                    # "Adding or removing from the array if there are active channels or not"
                    n85 = case shown="False" w620 {
                      tunnel: w613 -> [w627 w644]
                      tunnel: [w626 w641] -> w615
                      tunnel: [w625 w642] -> w616
                      tunnel: w617 -> [w624 w639]
                      tunnel: w614 -> [w623 w643]
                      tunnel: w619 -> [w622 w637]
                      tunnel: w618 -> [w621 w645]
                      frame False {
                        # "There are active channels"
                        n86 = case shown="False" w627 {
                          tunnel: w621 -> [w630 w636]
                          tunnel: w622 -> [w629 w635]
                          tunnel: w623 -> [_ w634]
                          tunnel: w624 -> [w631 w633]
                          tunnel: [w631 w633] -> w625
                          tunnel: [w628 w632] -> w626
                          frame False {
                            # "Instantiating the instrument into the array of instruments"
                            n87 = Insert Into Array(array=w630, new element=w629) -> (w628:T1)  [unwired: 1 in]
                          }
                          frame True {
                            # "Updating the instrument with the new configuration"
                            n88 = Replace Array Subset(array=w636, new element=w635, index=w634) -> (w632:T1)
                          }
                        }
                      }
                      frame True {
                        # "No active channels on the instrument currently"
                        n89 = Unbundle(w637) -> ("IVI Refnum out"=w640:refnum<k15>)  [unwired: 7 out]
                        n90 = call <instrlib>:"niDCPower Close.vi"("error in (no error)"=w639, "instrument handle"=w640) -> ("error out"=w638:errorcluster)  [unwired: 9 in]
                        n91 = case shown="True" w644 {
                          tunnel: w645 -> [w647 w651]
                          tunnel: w643 -> [_ w650]
                          tunnel: [w646 w649] -> w642
                          tunnel: w638 -> [w646 w649]
                          tunnel: [w647 w648] -> w641
                          frame False {
                            # "The instrument wasn't active and it is still not being used"
                          }
                          frame True {
                            # "The instrument was active but now it is not being used"
                            n92 = Delete From Array(array=w651, index=w650) -> (array with subset deleted=w648:T1)  [unwired: 1 in, 1 out]
                          }
                        }
                      }
                    }
                  }
                  frame Enabled {
                    # "v4. not removing instances with non active channels in this stage this will be in the update block outside"
                    # "Updating or instantiating the DCPower array with channel information"
                    n93 = case shown="True" w652 {
                      tunnel: w657 -> [w661 w667]
                      tunnel: w658 -> [w660 w666]
                      tunnel: w653 -> [_ w665]
                      tunnel: w656 -> [w662 w664]
                      tunnel: [w662 w664] -> w655
                      tunnel: [w659 w663] -> w654
                      frame False {
                        # "Instantiating the instrument into the array of instruments"
                        n94 = Insert Into Array(array=w661, new element=w660) -> (w659:T1)  [unwired: 1 in]
                      }
                      frame True {
                        # "Updating the instrument with the new configuration"
                        n95 = Replace Array Subset(array=w667, new element=w666, index=w665) -> (w663:T1)
                      }
                    }
                  }
                  frame Disabled {
                    n96 = for {
                      tunnel: w672 -> [w678] mode=indexing
                      shift-right: [w677] -> w671
                      shift-left: w670 -> [w677]
                      tunnel: w669 -> [w675]
                      tunnel: FALSE -> [w673]
                      n97 = Unbundle By Name(w675) -> ("IVI Refnum out"=w674:refnum<k15>)
                      n98 = Unbundle By Name(w678) -> ("IVI Refnum out"=w676:refnum<k15>)
                      n99 = Equal?(x=w676, y=w674) -> ()  [unwired: 1 out]
                      n100 = case shown="True" w673 {
                        frame False {
                        }
                        frame True {
                        }
                      }
                    }
                  }
                }
              }
            }
          }
        }
      }
      frame "Slot_16_PXIe4139" {
        n101 = Build Array("Channel Name 0") -> (w686:string[])
        n102 = Build Array("Active Channel 0") -> (w687:bool[])
        n103 = Build Array("voltage level channel 25") -> (w688:dbl[])
        n104 = case shown="True" "Apply Power Settings" {
          tunnel: w681 -> [w696 w709]
          tunnel: refnum<k15> "Slot_16_PXIe4139" ("resource name") -> [_ w698]
          tunnel: w687 -> [_ w724]
          tunnel: w686 -> [_ w722]
          tunnel: w689 -> [w695 w697]
          tunnel: [w695 w707] -> w683
          tunnel: [w696 w706] -> w684
          tunnel: w688 -> [_ w723]
          tunnel: [w694 FALSE] -> w680
          tunnel: w679 -> [w694 _]
          frame False {
          }
          frame True {
            # "This is the main block here: Takes the channels that are active, their voltages, and user defined name to determine the active channels on the instrument which is compared to the initial instrument array that is passed through it. The device capture time, current limit, record length are also configured here. This outputs the parameters of all channels, their voltages, names, if active, their current limit, and the time between records. This data will be put into a cluster which is then put into an array of DCPower Instruments. This array of instruments will be used to sample DUTs especially for latchup testing. These parameters will be recorded in a output config csv in a later part of the overall project."
            # "Checking if there are any active channels in this instrument"
            # "Could I have put all of this into a subVI? Yes. I didn't though because I didn't have an elegant way to make this into a type def based on each instrument having a different number of channels. Can go into the instrument config and make another subVI that creates another parameter of interest"
            # "Can't make a type def for this unless I do something elaborate for the toggling of channels active which I don't think I can do because each instrument has a different  number of channels which doesn't lend itself to making a type def"
            # "Test if this works properly"
            n105 = call "DCPower_ConfigureInstrument.vi"("IVI Refnum in"=w698, "current limit"="current limit (A)", "Aperture Time"="Aperture Time (s)", "Measure Record Length"="Measure Record Length", "Active Channels Input"=w724, "Channel Name Array"=w722, "error in (no error)"=w697, "Voltage Array Input"=w723, "DCPowerInformationClusterArray_Input"=w709) -> ("Active Channels Indicator"=→"Active Channels Indicator":bool[], "All Channel Numbers Array"=w700:string[], "Total Voltage Indicator Array"=→"Voltage Array":dbl[], "Active Channel Numbers String List"=w701:string, "IVI Ref index"=w705:i32, "IVI Refnum out"=w717:refnum<k15>, "Active Channel Numbers Array"=w703:string[], "Active Channel Names Array"=w715:string[], "Active Channel Current Limit Array"=w714:dbl[], "Active Channel Measure Record Delta Time Array"=w713:dbl[], "Active Channel Voltage Array"=w716:dbl[], "IVI Ref Present?"=w704:bool, "error out"=w708:errorcluster)  [unwired: 5 in, 1 out]
            "All Channel Numbers Array" <- w700
            "Active Channel Numbers Array" <- w703
            "Active Channel Names Array" <- w715
            "Active Channel Voltage Array" <- w716
            n106 = Bundle("IVI Refnum out"=w717, "Active Channel Numbers String List"=w701, "Active Channel Numbers Array"=w703, "Active Channel Voltage Array"=w716, "Active Channel Names Array"=w715, "Active Channel Current Limit Array"=w714, "Active Channel Measure Record Delta Time Array"=w713, "All Channel Numbers Array"=w700) -> (w710:T8)  [unwired: 1 in]
            n107 = Equal?(x=w701, y="") -> (x = y?=w711:bool)
            n108 = disable-structure shown="Enabled" {
              disable-tunnel: w711 -> [w732 w766]
              disable-tunnel: w710 -> [w731 w770]
              disable-tunnel: w709 -> [w730 w771]
              disable-tunnel: w708 -> [w729 w767]
              disable-tunnel: [w728 w765] -> w707
              disable-tunnel: [w727 w764] -> w706
              disable-tunnel: w705 -> [w726 w769]
              disable-tunnel: w704 -> [w725 w768]
              frame Disabled {
                # "Adding or removing from the array if there are active channels or not"
                n109 = case shown="False" w732 {
                  tunnel: w725 -> [w739 w756]
                  tunnel: [w738 w753] -> w727
                  tunnel: [w737 w754] -> w728
                  tunnel: w729 -> [w736 w751]
                  tunnel: w726 -> [w735 w755]
                  tunnel: w731 -> [w734 w749]
                  tunnel: w730 -> [w733 w757]
                  frame False {
                    # "There are active channels"
                    n110 = case shown="True" w739 {
                      tunnel: w733 -> [w742 w748]
                      tunnel: w734 -> [w741 w747]
                      tunnel: w735 -> [_ w746]
                      tunnel: w736 -> [w743 w745]
                      tunnel: [w743 w745] -> w737
                      tunnel: [w740 w744] -> w738
                      frame False {
                        # "Instantiating the instrument into the array of instruments"
                        n111 = Insert Into Array(array=w742, new element=w741) -> (w740:T1)  [unwired: 1 in]
                      }
                      frame True {
                        # "Updating the instrument with the new configuration"
                        n112 = Replace Array Subset(array=w748, new element=w747, index=w746) -> (w744:T1)
                      }
                    }
                  }
                  frame True {
                    # "No active channels on the instrument currently"
                    n113 = Unbundle(w749) -> ("IVI Refnum out"=w752:refnum<k15>)  [unwired: 7 out]
                    n114 = call <instrlib>:"niDCPower Close.vi"("error in (no error)"=w751, "instrument handle"=w752) -> ("error out"=w750:errorcluster)  [unwired: 9 in]
                    n115 = case shown="False" w756 {
                      tunnel: w757 -> [w759 w763]
                      tunnel: w755 -> [_ w762]
                      tunnel: [w758 w761] -> w754
                      tunnel: w750 -> [w758 w761]
                      tunnel: [w759 w760] -> w753
                      frame False {
                        # "The instrument wasn't active and it is still not being used"
                      }
                      frame True {
                        # "The instrument was active but now it is not being used"
                        n116 = Delete From Array(array=w763, index=w762) -> (array with subset deleted=w760:T1)  [unwired: 1 in, 1 out]
                      }
                    }
                  }
                }
              }
              frame Enabled {
                n117 = disable-structure shown="Enabled" {
                  disable-tunnel: w766 -> [w779 _ _]
                  disable-tunnel: w770 -> [w778 w817 w828]
                  disable-tunnel: w771 -> [w777 w816 w831]
                  disable-tunnel: w767 -> [w776 w815 w829]
                  disable-tunnel: [w775 w814 w830] -> w765
                  disable-tunnel: [w774 w813 _] -> w764
                  disable-tunnel: w769 -> [w773 w812 _]
                  disable-tunnel: w768 -> [w772 w811 _]
                  frame Disabled {
                    # "Original (v3) version where the array had only active channels"
                    # "Adding or removing from the array if there are active channels or not"
                    n118 = case shown="False" w779 {
                      tunnel: w772 -> [w786 w803]
                      tunnel: [w785 w800] -> w774
                      tunnel: [w784 w801] -> w775
                      tunnel: w776 -> [w783 w798]
                      tunnel: w773 -> [w782 w802]
                      tunnel: w778 -> [w781 w796]
                      tunnel: w777 -> [w780 w804]
                      frame False {
                        # "There are active channels"
                        n119 = case shown="False" w786 {
                          tunnel: w780 -> [w789 w795]
                          tunnel: w781 -> [w788 w794]
                          tunnel: w782 -> [_ w793]
                          tunnel: w783 -> [w790 w792]
                          tunnel: [w790 w792] -> w784
                          tunnel: [w787 w791] -> w785
                          frame False {
                            # "Instantiating the instrument into the array of instruments"
                            n120 = Insert Into Array(array=w789, new element=w788) -> (w787:T1)  [unwired: 1 in]
                          }
                          frame True {
                            # "Updating the instrument with the new configuration"
                            n121 = Replace Array Subset(array=w795, new element=w794, index=w793) -> (w791:T1)
                          }
                        }
                      }
                      frame True {
                        # "No active channels on the instrument currently"
                        n122 = Unbundle(w796) -> ("IVI Refnum out"=w799:refnum<k15>)  [unwired: 7 out]
                        n123 = call <instrlib>:"niDCPower Close.vi"("error in (no error)"=w798, "instrument handle"=w799) -> ("error out"=w797:errorcluster)  [unwired: 9 in]
                        n124 = case shown="True" w803 {
                          tunnel: w804 -> [w806 w810]
                          tunnel: w802 -> [_ w809]
                          tunnel: [w805 w808] -> w801
                          tunnel: w797 -> [w805 w808]
                          tunnel: [w806 w807] -> w800
                          frame False {
                            # "The instrument wasn't active and it is still not being used"
                          }
                          frame True {
                            # "The instrument was active but now it is not being used"
                            n125 = Delete From Array(array=w810, index=w809) -> (array with subset deleted=w807:T1)  [unwired: 1 in, 1 out]
                          }
                        }
                      }
                    }
                  }
                  frame Enabled {
                    # "v4. not removing instances with non active channels in this stage this will be in the update block outside"
                    # "Updating or instantiating the DCPower array with channel information"
                    n126 = case shown="True" w811 {
                      tunnel: w816 -> [w820 w826]
                      tunnel: w817 -> [w819 w825]
                      tunnel: w812 -> [_ w824]
                      tunnel: w815 -> [w821 w823]
                      tunnel: [w821 w823] -> w814
                      tunnel: [w818 w822] -> w813
                      frame False {
                        # "Instantiating the instrument into the array of instruments"
                        n127 = Insert Into Array(array=w820, new element=w819) -> (w818:T1)  [unwired: 1 in]
                      }
                      frame True {
                        # "Updating the instrument with the new configuration"
                        n128 = Replace Array Subset(array=w826, new element=w825, index=w824) -> (w822:T1)
                      }
                    }
                  }
                  frame Disabled {
                    n129 = for {
                      tunnel: w831 -> [w837] mode=indexing
                      shift-right: [w836] -> w830
                      shift-left: w829 -> [w836]
                      tunnel: w828 -> [w834]
                      tunnel: FALSE -> [w832]
                      n130 = Unbundle By Name(w834) -> ("IVI Refnum out"=w833:refnum<k15>)
                      n131 = Unbundle By Name(w837) -> ("IVI Refnum out"=w835:refnum<k15>)
                      n132 = Equal?(x=w835, y=w833) -> ()  [unwired: 1 out]
                      n133 = case shown="True" w832 {
                        frame False {
                        }
                        frame True {
                        }
                      }
                    }
                  }
                }
              }
            }
          }
        }
      }
    }
    "VISAPowerInformationClusterArray" <- w26
    "Supplies Updated?" <- w14
    n134 = case shown="True" "Update Changes (MUST HAVE ACTIVE CHANNEL SELECTED FOR CHANGES TO BE APPLIED)" {
      selector: "Update Changes (MUST HAVE ACTIVE CHANNEL SELECTED FOR CHANGES TO BE APPLIED)" -> [_ w51]
      tunnel: [w30 w43] -> w9
      tunnel: w17 -> [w30 w53]
      tunnel: w15 -> [w31 w52]
      tunnel: [w31 w42] -> w8
      tunnel: w14 -> [w29 _]
      tunnel: [w29 w51] -> w12
      frame False {
      }
      frame True {
        # "Fetching some data to confirm part is powered on properly. Indicators are shown to the right"
        # "Making all the colors and names of the chart \"none\" so empty names are called \"none\""
        # "renaming the legend and the colors of the chart"
        # "closing the instrument if it is not configured anymore"
        n135 = for {
          tunnel: [w105] -> w43 mode=indexing if=w93
          tunnel: w53 -> [w105] mode=indexing
          shift-right: [w95] -> w48
          shift-left: w52 -> [w103]
          n136 = Unbundle(w105) -> ("IVI Refnum out"=w104:refnum<k15>, "Active Channel Numbers String List"=w99:string, "All Channel Numbers Array"=w98:string[])  [unwired: 5 out]
          n137 = Equal?(x=w99, y="") -> (x = y?=w94:bool)
          n138 = call "StringArray2StringList.vi"("String Array"=w98) -> ("String List"=w97:string)
          n139 = call <instrlib>:"niDCPower Initiate With Channels.vi"("error in (no error)"=w103, "channel name"=w97, "instrument handle"=w104) -> ("error out"=w102:errorcluster, "instrument handle out"=w101:refnum<k15>)  [unwired: 7 in]
          n140 = call <instrlib>:"niDCPower Abort With Channels.vi"("error in (no error)"=w102, "channel name"=w97, "instrument handle"=w101) -> ("error out"=w96:errorcluster, "instrument handle out"=w92:refnum<k15>)  [unwired: 7 in]
          n141 = case shown="True" w94 {
            tunnel: w96 -> [w106 w109]
            tunnel: [w106 w107] -> w95
            tunnel: w92 -> [_ w108]
            frame False {
            }
            frame True {
              n142 = call <instrlib>:"niDCPower Close.vi"("error in (no error)"=w109, "instrument handle"=w108) -> ("error out"=w107:errorcluster)  [unwired: 9 in]
            }
          }
          n143 = Not(x=w94) -> (.not. x?=w93:bool)
        }
        "DCPowerInformationClusterArray" <- w43
        n144 = for {
          tunnel: w43 -> [w91] mode=indexing
          shift-right: [w88] -> w49
          shift-left: w48 -> [w87]
          n145 = Unbundle By Name(w91) -> ("IVI Refnum out"=w89:refnum<k15>, "Active Channel Numbers String List"=w90:string)
          n146 = call <instrlib>:"niDCPower Initiate With Channels.vi"("error in (no error)"=w87, "channel name"=w90, "instrument handle"=w89) -> ("error out"=w88:errorcluster)  [unwired: 7 in, 1 out]
        }
        n147 = call "Convert_InstrumentReferenceArray_2_ChannelReferenceArray.vi"("error in (no error)"=w49, "DCPowerInformationClusterArray_Input"=w43) -> ("error out"=w46:errorcluster, "DCPowerInformation_byChannel"=w45:T9)
        n148 = for {
          shift-right: [w80] -> w47
          shift-left: w46 -> [w78]
          tunnel: "ColorPalette" -> [_] mode=indexing
          i -> [w77]
          w76 = "NONE" ("Plot.Plot Name")
          n149 = property on="Current Waveform Array" class="WFChart (strict)"(error in=w78, "Active Plot"=w77, "Plot.Plot Name"=w76) -> (error out=w79:errorcluster)  [unwired: 1 in, 1 out]
          n150 = property on="Voltage Waveform Array" class="WFChart (strict)"(error in=w79, "Active Plot"=w77, "Plot.Plot Name"=w76) -> (error out=w80:errorcluster)  [unwired: 1 in, 1 out]
        }
        n151 = case shown="No Error" w47 {
          selector: w47 -> [w74 _]
          tunnel: [w74 w75] -> w40
          tunnel: w46 -> [_ w75]
          frame No Error {
          }
          frame Error {
          }
        }
        n152 = for {
          shift-right: [w71] -> w39
          shift-left: w40 -> [w72]
          tunnel: w45 -> [w70] mode=indexing
          tunnel: "ColorPalette" -> [w69] mode=indexing
          tunnel: "ColorPalette" -> [w68] mode=indexing
          i -> [w67]
          n153 = Unbundle By Name(w70) -> ("Channel Name 23"=w66:string)
          n154 = property on="Current Waveform Array" class="WFChart (strict)"(error in=w72, "Active Plot"=w67, "Plot.Plot Name"=w66, "Plot.Plot Color"=w69) -> (error out=w73:errorcluster)  [unwired: 1 in, 1 out]
          n155 = property on="Voltage Waveform Array" class="WFChart (strict)"(error in=w73, "Active Plot"=w67, "Plot.Plot Name"=w66, "Plot.Plot Color"=w68) -> (error out=w71:errorcluster)  [unwired: 1 in, 1 out]
        }
        n156 = case shown="Error .." w39 {
          selector: w39 -> [w59 _]
          tunnel: [w59 w60] -> w41
          tunnel: w40 -> [_ w60]
          frame No Error {
          }
          frame Error {
          }
        }
        n157 = for {
          N: 1000 -> [_]
          tunnel: w45 -> [w86]
          tunnel: timestamp(0 s since 1904-01-01) ("Initial Time") -> [w85]
          shift-right: [w83] -> w36
          shift-left: w41 -> [w84]
          tunnel: [w82] -> w38
          tunnel: [w81] -> w35
          n158 = call "Fetch&Process_Measurements_V4.vi"("DCPowerInformation_byChannel"=w86, "Initial Time"=w85, "error in (no error)"=w84) -> ("Current Waveform Array"=w81:waveform(dbl)[], "Voltage Waveform Array"=w82:waveform(dbl)[], "error out"=w83:errorcluster)  [unwired: 6 in, 4 out]
          "Current Waveform Array" <- w81
          "Voltage Waveform Array" <- w82
        }
        n159 = for {
          tunnel: w38 -> [w58] mode=indexing
          shift-right: [w57] -> w37
          shift-left: w36 -> [w57]
          tunnel: w35 -> [w56] mode=indexing
          tunnel: [w55] -> w34 mode=indexing
          tunnel: [w54] -> w33 mode=indexing
          n160 = Unbundle By Name(w56) -> ("Y"=w54:dbl[])
          n161 = Unbundle By Name(w58) -> ("Y"=w55:dbl[])
        }
        "Voltage Numeric (V)" <- w34
        "Current Numeric (A)" <- w33
        n162 = for {
          tunnel: w43 -> [w65] mode=indexing
          shift-right: [w61] -> w42
          shift-left: w37 -> [w62]
          n163 = Unbundle By Name(w65) -> ("IVI Refnum out"=w64:refnum<k15>, "Active Channel Numbers String List"=w63:string)
          n164 = call <instrlib>:"niDCPower Abort With Channels.vi"("error in (no error)"=w62, "channel name"=w63, "instrument handle"=w64) -> ("error out"=w61:errorcluster)  [unwired: 7 in, 1 out]
        }
      }
    }
    n165 = Array Size(array=w17) -> (size(s)=w25:i32)
    n166 = Array Size(array=w26) -> (size(s)=w24:i32)
    n167 = Not Equal To 0?(x=w25) -> (x != 0?=w22:bool)
    n168 = Not Equal To 0?(x=w24) -> (x != 0?=w23:bool)
    n169 = Or(x=w22, y=w23) -> (x .or. y?=w20:bool)
    n170 = case shown="True" "Exit SubVI" {
      selector: "Exit SubVI" -> [w110 w114]
      tunnel: w20 -> [_ w112]
      tunnel: [w110 w115] -> w19
      tunnel: w12 -> [_ w111]
      frame False {
      }
      frame True {
        n171 = And(x=w111, y=w112) -> (x .and. y?=w113:bool)
        n172 = case shown="False" w113 {
          tunnel: [w117 w120] -> w115
          tunnel: w114 -> [_ w120]
          frame False {
            n173 = Two Button Dialog(message="You need to have at least one channel configured and updated", 1:"Ok, I will stay in this VI" ("F button name (\"Cancel\")"), 2:"No, screw off, I'm exiting this VI without a channel configured" ("T button name (\"OK\")")) -> (T button?=w117:bool)
          }
          frame True {
          }
        }
      }
    }
    n174 = Or(x=w8, y=w19) -> (x .or. y?=w18:bool)
  }
  "error out" <- w6
  "VISAPowerInfoOutputArray" <- w4
  "DCPowerInformationClusterArray_Output" <- w3
  n175 = disable-structure shown="Disabled" {
    disable-tunnel: _ -> [w839 _]
    disable-tunnel: _ -> [w838 _]
    frame Disabled {
      n176 = for {
        shift-right: [w840] -> _
        shift-left: w839 -> [w843]
        tunnel: w838 -> [w842] mode=indexing
        n177 = Unbundle(w842) -> ("instrument handle out"=w841)  [unwired: 4 out]
        n178 = call <instrlib>:"niDCPower Close.vi"("error in (no error)"=w843, "instrument handle"=w841) -> ("error out"=w840:errorcluster)  [unwired: 9 in]
      }
    }
    frame Enabled {
    }
  }
